vi "Set Boolean.vi"(8 "error in (no error)":errorcluster, 10 "Boolean":bool, 11 "JSON Scalar in":refnum<class "JSON Scalar.lvclass">) -> (0 "error out":errorcluster, 3 "JSON Scalar out":refnum<class "JSON Scalar.lvclass">)   [LabVIEW 2020, in "Library Commun.lvlib" / "JSON Scalar.lvclass"]
doc: "Stores a <b>Boolean</b> as a <b>JSON Scalar</b>.\n\nCopyright 2012 James David Powell, Shaun Rumbell and Ton Plomp\nMore information on http://lavag.org/topic/16217-cr-json-labview"
uses:
  JSON Scalar.lvclass
  JSON Scalar.lvclass/JSON Scalar.ctl
  Quote and Escape JSON string.vi
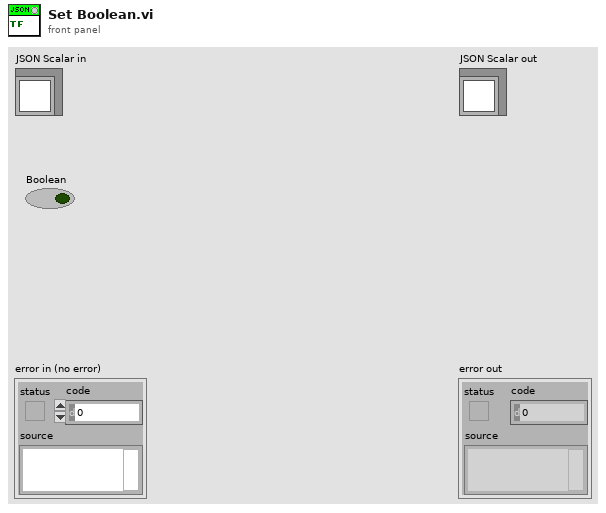
[diagram p1: front panel]
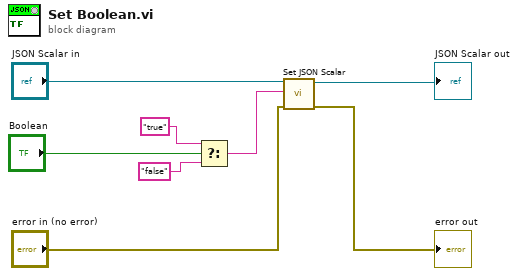
[diagram p0: block diagram]
diagram:
  n1 = Select(t="true", s="Boolean", f="false") -> (s? t:f=w2:string)
  n2 = call "Set JSON Scalar.vi"("error in (no error)"="error in (no error)", "LabVIEW Text"=w2, "JSON Scalar in"="JSON Scalar in") -> ("error out"=→"error out":errorcluster, "JSON Scalar out"=→"JSON Scalar out":refnum<class "JSON Scalar.lvclass">)  [unwired: 7 in]
